vi "Bus Interface.vi"(0 "niUSRP Tx DSP v2 FPGA":refnum<class "niUSRP Tx DSP v2 FPGA.lvclass">, 1 "abort":bool, 5 "instruction":T2, 9 "input valid":bool) -> (6 "response":T1, 10 "done":bool, 14 "ready for input":bool)   [LabVIEW 2025, in "niUSRP Tx DSP v2 FPGA.lvclass"]
uses:
  niUSRP Tx DSP v2 FPGA.lvclass
  <instrlib>/_niInstr/Instruction Framework/v1/FPGA/Interfaces/Address Space/Address Space Instruction.ctl
  <instrlib>/_niInstr/Instruction Framework/v1/FPGA/Typedefs/Response.ctl
  niUSRP Tx DSP v2 FPGA.lvclass/niUSRP Tx DSP v2 FPGA.ctl
  <vilib>/rvi/DataTransferAndStorage/Container/Common/niFpgaContainerExecOnDevCompGetState.vi
  <vilib>/rvi/Emulation/niFpgaEmulationIsFPGAContextNoSignature.vi
  <vilib>/rvi/DataTransferAndStorage/Container/Common/niFpgaContainerGetUniqueNameForEmu.vi
  <vilib>/rvi/Memory/Memory_Emulation/niFpgaMemoryEmulationCacheClearOnFirstRun.vi
  <vilib>/rvi/Memory/Memory_Emulation/nirvimemoryEmulationManagerCache_MakeExclusive.vi
  <vilib>/rvi/Memory/Memory_Emulation/niFpgaMemoryEmulationValidateCache.vi
  <vilib>/rvi/Memory/Memory_Emulation/nirvimemoryEmulationManagerCache_InsertValue.vi
  <vilib>/Utility/error.llb/Clear Errors.vi
  <vilib>/rvi/Memory/Memory_Emulation/nirvimemoryEmulationManagerCache_ReleaseExclusive.vi
  <vilib>/rvi/Memory/Memory_Emulation/nirvimemoryEmulationManagerCache_GetValue.vi
  <vilib>/rvi/Memory/Memory_Emulation/nirvimemoryEmulationManagerCache_SetValue.vi
  <vilib>/rvi/Emulation/niFpgaProcessEmulError.vi
  <vilib>/rvi/Emulation/niFpgaSctlEmulationGetInTimedLoop.vi
  <vilib>/rvi/DataTransferAndStorage/Container/XNode/niFpgaContainer.xnode
  <vilib>/rvi/DataTransferAndStorage/Register/Emulation/niFpgaRegisterEmulationRefIn.vi
  <instrlib>/_niInstr/Instruction Framework/v1/FPGA/Typedefs/niInstr Instruction Framework v1 FPGA.lvlib
  <instrlib>/_niInstr/Instruction Framework/v1/FPGA/Interfaces/Address Space/Address Space.lvclass
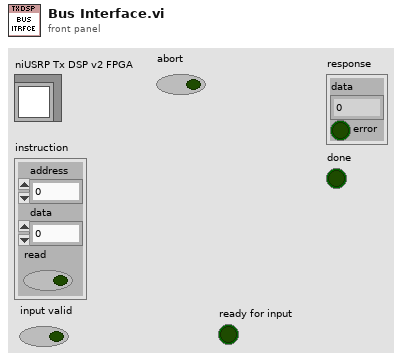
[diagram p1: front panel]
types:
  T1 = typedef "niInstr Instruction Framework v1 FPGA.lvlib/Response.ctl" = cluster{"data":u64, "error":bool}
  T2 = typedef "niInstr Instruction Framework Interfaces v1 FPGA.lvlib/Address Space.lvclass/Address Space Instruction.ctl" = cluster{"address":u32, "data":u64, "read":bool}
  T3 = typedef "niUSRP Tx DSP v2 FPGA.lvclass/Tx DSP Shared Registers.ctl" = cluster{"reset":refnum<k21>, "reset.done":refnum<k21>, "ignore overflows":refnum<k21>, "overflow":refnum<k21>, "overflow.clear":refnum<k21>, "pipeline delay":refnum<k21>, "group delay (output samples)":refnum<k21>, "blanking delay.data clock ticks":refnum<k21>, "dynamic delay.data clock ticks":refnum<k21>, "dynamic delay.samples":refnum<k21>, "bypass EQ":refnum<k21>, "inject idle into path":refnum<k21>, "TxDspEnabled":refnum<k21>}
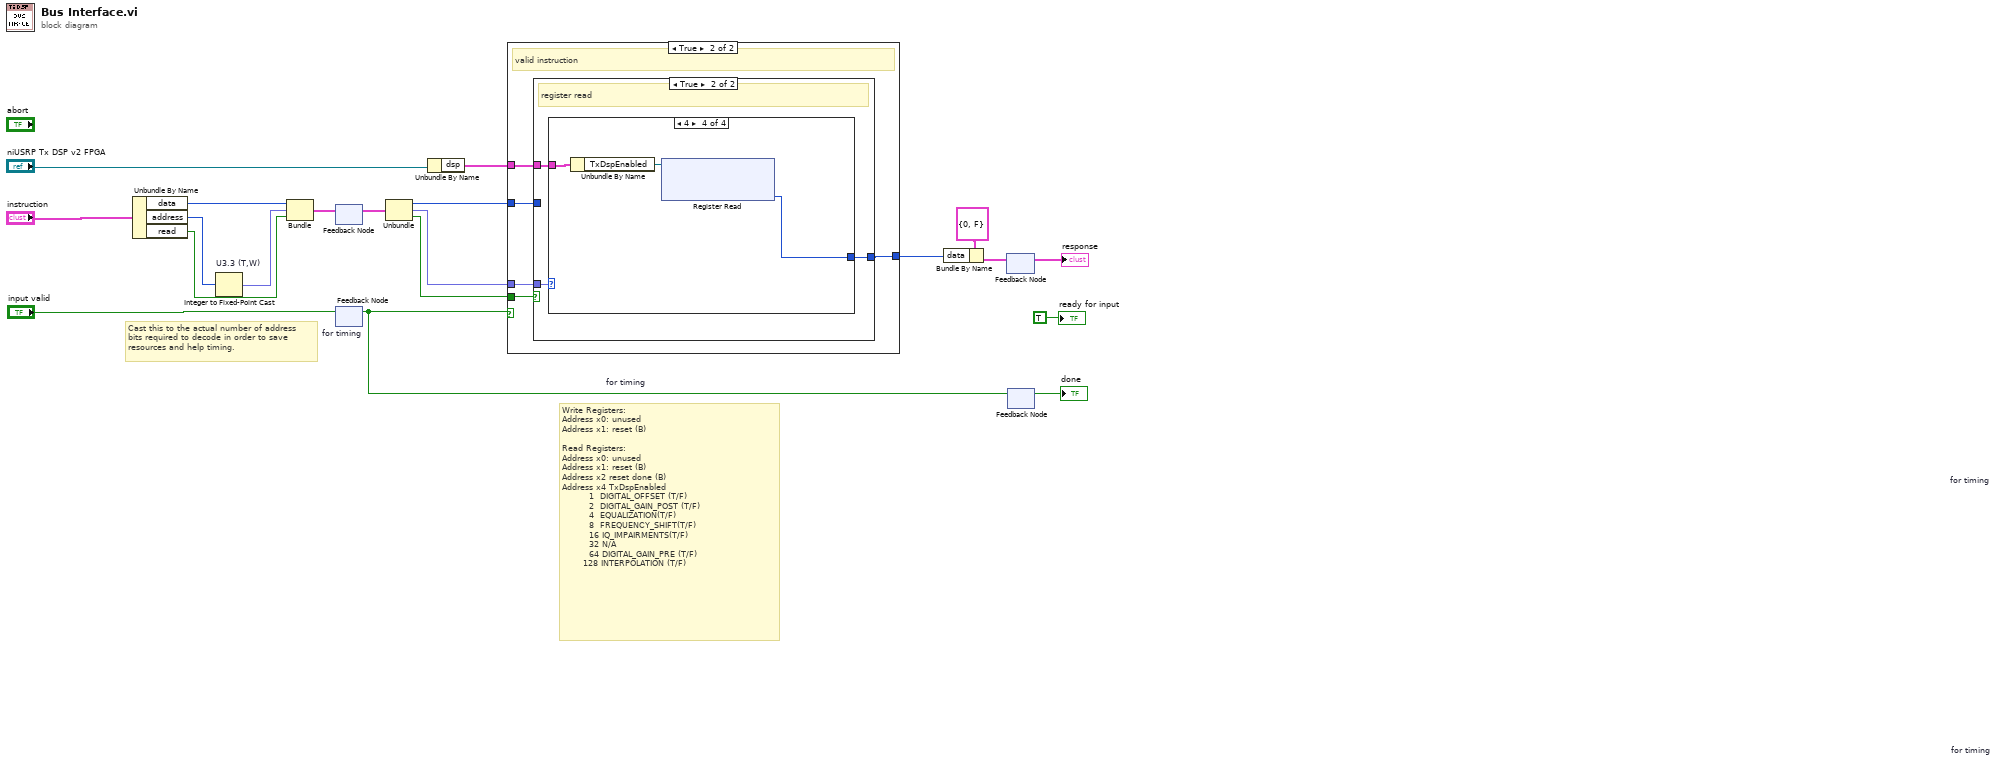
[diagram p0: block diagram]
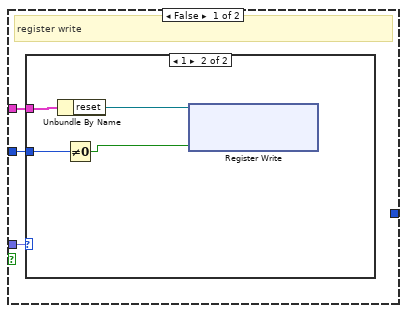
[diagram p3: hidden frame]
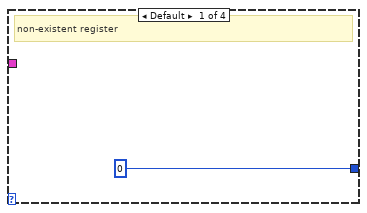
[diagram p5: hidden frame]
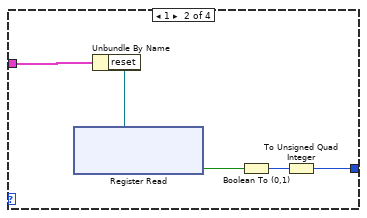
[diagram p6: hidden frame]
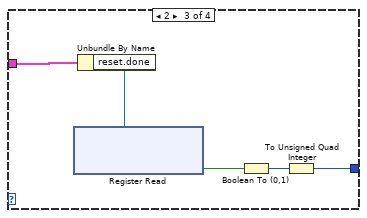
[diagram p7: hidden frame]
diagram:
  # "Write Registers:\nAddress x0: unused\nAddress x1: reset (B)\n\nRead Registers:\nAddress x0: unused\nAddress x1: reset (B)\nAddress x2 reset done (B)\nAddress x4 TxDspEnabled\n         1  DIGITAL_OFFSET (T/F)\n         2  DIGITAL_GAIN_POST (T/F)\n         4  EQUALIZATION(T/F)\n         8  FREQUENCY_SHIFT(T/F)\n         16 IQ_IMPAIRMENTS(T/F)\n         32 N/A\n         64 DIGITAL_GAIN_PRE (T/F)\n       128 INTERPOLATION (T/F)"
  # "Cast this to the actual number of address\nbits required to decode in order to save\nresources and help timing."
  n1 = Unbundle By Name("instruction") -> ("data"=w17:u64, "address"=w20:u32, "read"=w15:bool)
  n2 = Integer to Fixed-Point Cast "U3.3 (T,W)"(integer=w20) -> (fixed-point=w16:fxp<+,3,3>)  [unwired: 1 in]
  n3 = Bundle("data"=w17, w16, "read"=w15) -> (w19:cluster{"data":u64, fxp<+,3,3>, "read":bool})  [unwired: 1 in]
  n4 = feedback #1 "for timing"() -> (w18:cluster{"data":u64, fxp<+,3,3>, "read":bool})  [unwired: 1 in]
  n5 = feedback-in #1(w19) -> ()
  n6 = feedback #2 "for timing"() -> (w7:bool)  [unwired: 1 in]
  n7 = feedback-in #2("input valid") -> ()
  n8 = Unbundle(w18) -> ("data"=w11:u64, w12:fxp<+,3,3>, "read"=w13:bool)
  n9 = Unbundle By Name("niUSRP Tx DSP v2 FPGA") -> ("dsp"=w14:T3)
  n10 = case shown="True" w7 {
    tunnel: w14 -> [_ w25]
    tunnel: w13 -> [_ w24]
    tunnel: w12 -> [_ w23]
    tunnel: w11 -> [_ w22]
    tunnel: [_ w21] -> w10
    frame False {
      # "invalid instruction"
    }
    frame True {
      # "valid instruction"
      n11 = case shown="True" w24 {
        tunnel: w23 -> [w28 w35]
        tunnel: [_ w33] -> w21
        tunnel: w22 -> [w27 _]
        tunnel: w25 -> [w26 w34]
        frame False {
          # "register write"
          n12 = case shown="1" w28 {
            tunnel: w27 -> [_ w29]
            tunnel: w26 -> [_ w30]
            frame Default {
              # "non-existent register"
            }
            frame 1 {
              n13 = Unbundle By Name(w30) -> ("reset"=w31:refnum<k21>)
              n14 = Not Equal To 0?(x=w29) -> (x != 0?=w32:bool)
              n15 = xnode ("Register Write")("Data"=w32, "Register In"=w31) -> ()  [unwired: 1 out]
            }
          }
        }
        frame True {
          # "register read"
          n16 = case shown="4" w35 {
            tunnel: w34 -> [_ w39 w44 w49]
            tunnel: [u64 0 w41 w46 w47] -> w33
            frame Default {
              # "non-existent register"
            }
            frame 1 {
              n17 = Unbundle By Name(w39) -> ("reset"=w40:refnum<k21>)
              n18 = xnode ("Register Read")("Register In"=w40) -> ("Data"=w38:bool)  [unwired: 1 out]
              n19 = Boolean To (0,1)(Boolean=w38) -> (0, 1=w37:i16)
              n20 = To Unsigned Quad Integer(1:w37) -> (0:w41:u64)
            }
            frame 2 {
              n21 = Unbundle By Name(w44) -> ("reset.done"=w45:refnum<k21>)
              n22 = xnode ("Register Read")("Register In"=w45) -> ("Data"=w43:bool)  [unwired: 1 out]
              n23 = Boolean To (0,1)(Boolean=w43) -> (0, 1=w42:i16)
              n24 = To Unsigned Quad Integer(1:w42) -> (0:w46:u64)
            }
            frame 4 {
              n25 = Unbundle By Name(w49) -> ("TxDspEnabled"=w48:refnum<k21>)
              n26 = xnode ("Register Read")("Register In"=w48) -> ("Data"=w47:u64)  [unwired: 1 out]
            }
          }
        }
      }
    }
  }
  n27 = Bundle By Name(cluster=T1 {"data"=0, "error"=FALSE} ("response"), "data"=w10) -> (w8:T1)
  n28 = feedback #3 "for timing"() -> (→"response":T1)  [unwired: 1 in]
  n29 = feedback-in #3(w8) -> ()
  n30 = feedback #4 "for timing"() -> (→"done":bool)  [unwired: 1 in]
  n31 = feedback-in #4(w7) -> ()
  "ready for input" <- TRUE ("ready for input")
